vi "Pockels Cal-Load pockels file by name.vi"(8 "error in":errorcluster, 11 "Pockels cal file name":string) -> (0 "error out":errorcluster, 3 "Pockels cal file name":string)   [LabVIEW 2013]
uses:
  Typedefs/Read Write Enum.ctl
  Typedefs/Functional global standard states.ctl
  Globals/gl_Calibration globals.vi
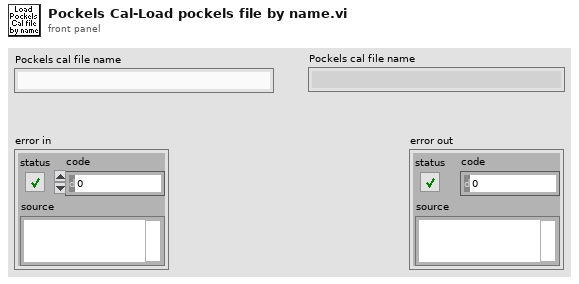
[diagram p1: front panel]
types:
  T1 = typedef "Functional global standard states.ctl" = enum16{"Initialise", "Read", "Write", "Load", "Save", "Clear"}
  T2 = typedef "Read Write Enum.ctl" = enum16{"Read", "Write"}
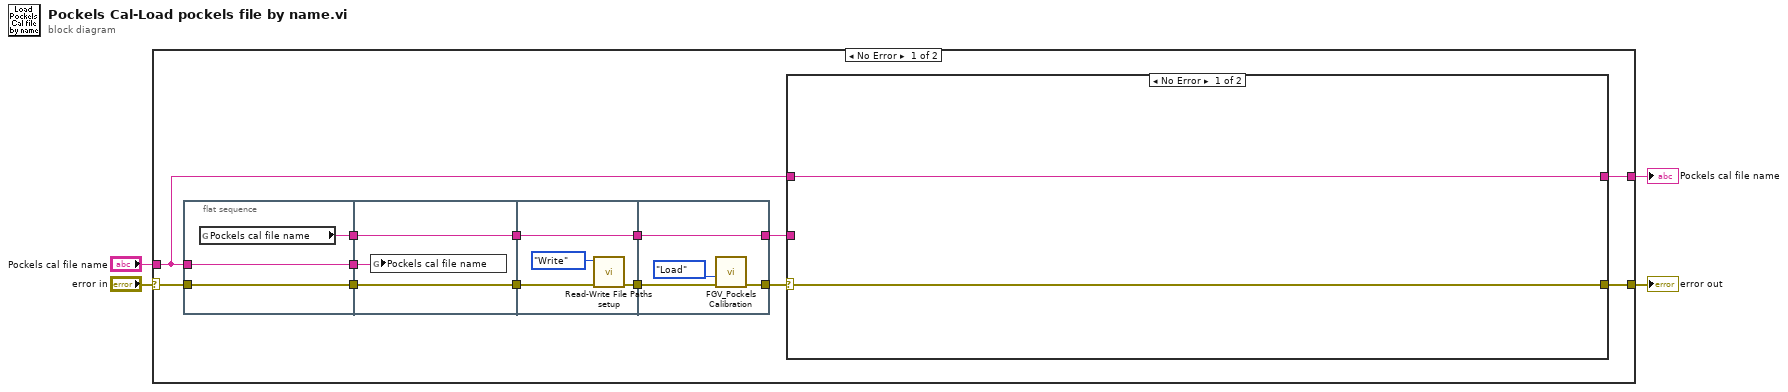
[diagram p0: block diagram]
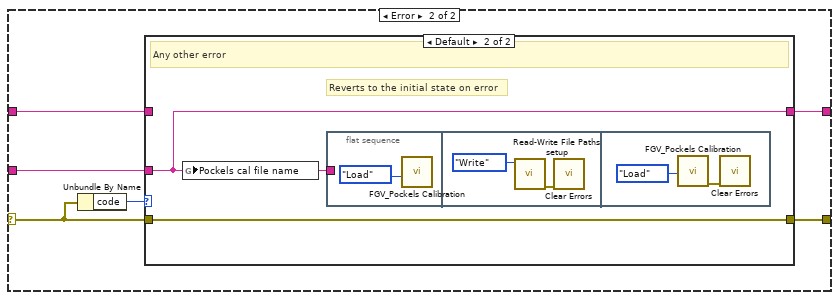
[diagram p2: hidden frame]
diagram:
  n1 = case shown="No Error" "error in" {
    selector: "error in" -> [w5 w49]
    tunnel: [w9 w49] -> w4
    tunnel: "Pockels cal file name" -> [w7 w48]
    tunnel: [w6 w48] -> w2
    frame No Error {
      n2 = flat-sequence {
        tunnel: w7 -> [w36]
        tunnel: [w36] -> w17
        tunnel: [w35] -> w16
        tunnel: [w34] -> w15
        tunnel: w5 -> [w34]
        tunnel: w17 -> [w39]
        tunnel: [w38] -> w14
        tunnel: w16 -> [w38]
        tunnel: [w37] -> w13
        tunnel: w15 -> [w37]
        tunnel: [w42] -> w12
        tunnel: [w41] -> w11
        tunnel: w14 -> [w41]
        tunnel: w13 -> [w40]
        tunnel: w12 -> [w46]
        tunnel: [w45] -> w10
        tunnel: [w44] -> w8
        tunnel: w11 -> [w44]
        frame #0 {
          n3 = global read "gl_Calibration globals.vi" "Pockels cal file name"() -> (w35:string)
        }
        frame #1 {
          n4 = global write "gl_Calibration globals.vi" "Pockels cal file name"(w39) -> ()
        }
        frame #2 {
          n5 = call "Read-Write File Paths setup.vi"("error in"=w40, "Function"=Read_Write_Enum."Write") -> ("error out"=w42:errorcluster)  [unwired: 9 in]
        }
        frame #3 {
          n6 = call "FGV_Pockels Calibration.vi"("error in (no error)"=w46, "Function"=Functional_global_standard_states."Load") -> ("error out"=w45:errorcluster)  [unwired: 3 in, 6 out]
        }
      }
      n7 = case shown="No Error" w10 {
        selector: w10 -> [w19 w23]
        tunnel: [w19 w22] -> w9
        tunnel: w8 -> [_ w25]
        tunnel: [w18 w21] -> w6
        tunnel: w7 -> [w18 w20]
        frame No Error {
        }
        frame Error {
          n8 = Unbundle By Name(w23) -> ("code"=w24:i32)
          n9 = case shown="Default" w24 {
            tunnel: w25 -> [_ w27]
            tunnel: w23 -> [_ w28]
            tunnel: [_ w28] -> w22
            tunnel: [w26 w27] -> w21
            tunnel: w20 -> [w26 _]
            frame 5003, 5004 {
              # "Default cal has been loaded"
            }
            frame Default {
              # "Reverts to the initial state on error"
              # "Any other error"
              n10 = global write "gl_Calibration globals.vi" "Pockels cal file name"(w27) -> ()
              n11 = flat-sequence {
                tunnel: w27 -> [_]
                frame #0 {
                  n12 = call "FGV_Pockels Calibration.vi"("Function"=Functional_global_standard_states."Load") -> ()  [unwired: 4 in, 7 out]
                }
                frame #1 {
                  n13 = call "Read-Write File Paths setup.vi"("Function"=Read_Write_Enum."Write") -> ("error out"=w30:errorcluster)  [unwired: 10 in]
                  n14 = call <vilib>:"Clear Errors.vi"("error in (no error)"=w30) -> ()  [unwired: 6 in, 1 out]
                }
                frame #2 {
                  n15 = call "FGV_Pockels Calibration.vi"("Function"=Functional_global_standard_states."Load") -> ("error out"=w32:errorcluster)  [unwired: 4 in, 6 out]
                  n16 = call <vilib>:"Clear Errors.vi"("error in (no error)"=w32) -> ()  [unwired: 6 in, 1 out]
                }
              }
            }
          }
        }
      }
    }
    frame Error {
    }
  }
  "error out" <- w4
  "Pockels cal file name" <- w2
